vi "ReadBulkPrePos.vi"(8 "error in":errorcluster) -> (0 "error out":errorcluster, 3 "Data":u8[](array[numeric]) format="%x")   [LabVIEW 2015]
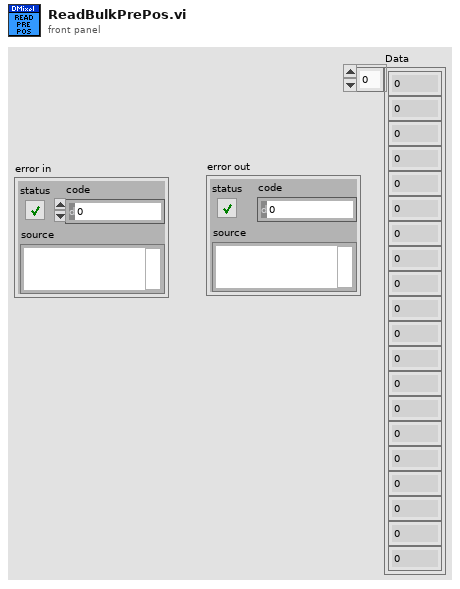
[diagram p1: front panel]
types:
  T1 = cluster{u8, u8, u8, u8, "x":u8, "x":u8, u8, "x":u8, "x":u8, u8, "x":u8, "x":u8, u8, "x":u8, "x":u8, u8, "x":u8, "x":u8, u8, "x":u8, "x":u8, u8}
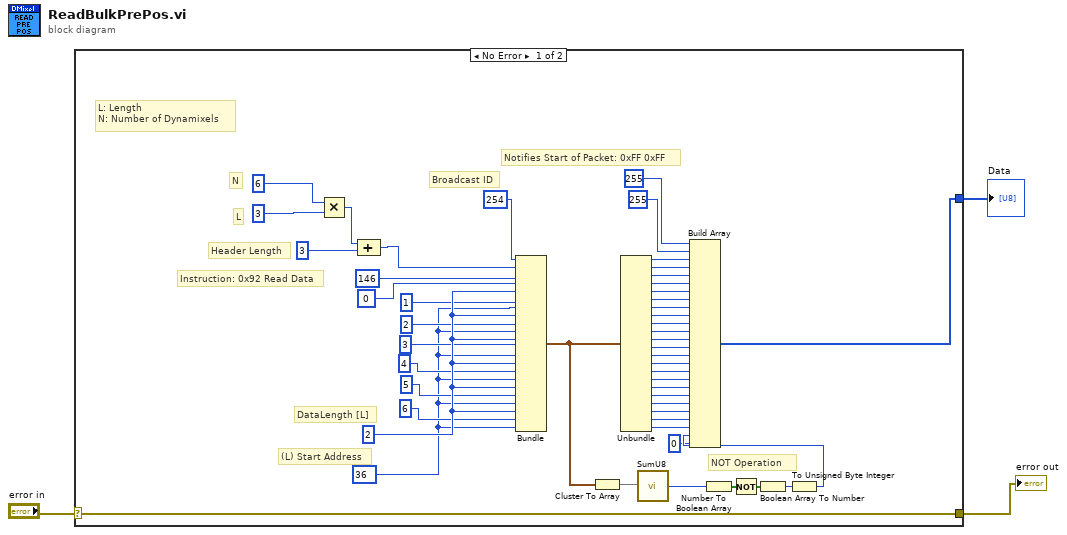
[diagram p0: block diagram]
diagram:
  n1 = case shown="No Error" "error in" {
    selector: "error in" -> [w5 _]
    tunnel: [w45 _] -> w2
    tunnel: [w5 _] -> w1
    frame No Error {
      w30 = u8 36
      w37 = u8 2 ("x")
      # "NOT Operation"
      # "DataLength [L]"
      # "L"
      # "L: Length \nN: Number of Dynamixels"
      # "Header Length"
      # "N"
      # "(L) Start Address"
      # "Instruction: 0x92 Read Data"
      # "Broadcast ID"
      # "Notifies Start of Packet: 0xFF 0xFF"
      n2 = Multiply(x=u8 6 ("N"), y=u8 3) -> (x*y=w53:u8)
      n3 = Compound Arithmetic op=unknown(w53, u8 3 ("value")) -> (w52:u8)
      n4 = Bundle(u8 254, w52, u8 146, u8 0, "x"=w37, "x"=u8 1, w30, "x"=w37, "x"=u8 2, w30, "x"=w37, "x"=u8 3, w30, "x"=w37, "x"=u8 4, w30, "x"=w37, "x"=u8 5, w30, "x"=w37, "x"=u8 6, w30) -> (w9:T1)  [unwired: 1 in]
      n5 = Cluster To Array(cluster=w9) -> (array=w8:u8[])
      n6 = Unbundle(w9) -> (w41:u8, w42:u8, w43:u8, w44:u8, "x"=w40:u8, "x"=w29:u8, w28:u8, "x"=w27:u8, "x"=w26:u8, w25:u8, "x"=w24:u8, "x"=w23:u8, w22:u8, "x"=w21:u8, "x"=w20:u8, w19:u8, "x"=w18:u8, "x"=w17:u8, w16:u8, "x"=w15:u8, "x"=w14:u8, w13:u8)
      n7 = call "SumU8.vi"("Array"=w8) -> ("Sum"=w7:u8)
      n8 = Number To Boolean Array(number=w7) -> (Boolean array=w10:bool[])
      n9 = Not(x=w10) -> (.not. x?=w11:bool[])
      n10 = Boolean Array To Number(Boolean array=w11) -> (number=w12:u8)
      n11 = To Unsigned Byte Integer(number=w12) -> (unsigned 8bit integer=w6:u8)
      n12 = Build Array(u8 255, u8 255, w41, w42, w43, w44, w40, w29, w28, w27, w26, w25, w24, w23, w22, w21, w20, w19, w18, w17, w16, w15, w14, w13, w6, u8 0 ("element")) -> (w45:u8[])
    }
    frame Error {
    }
  }
  "error out" <- w1
  "Data" <- w2
